vi "Set_Sweep_Frequency.vi"(8 "error in (no error)":errorcluster, 9 "endfreq":dbl, 10 "startfreq":dbl, 11 ".NET Reference in":refnum<k24>) -> (0 "error out":errorcluster, 3 "Reference out":refnum<k24>)   [LabVIEW 2017]
uses:
  D:/test/FULLband-sts/Fullband_Sample/DLL/InstrumentDLL.dll
  DLL/InstrumentDLL.dll
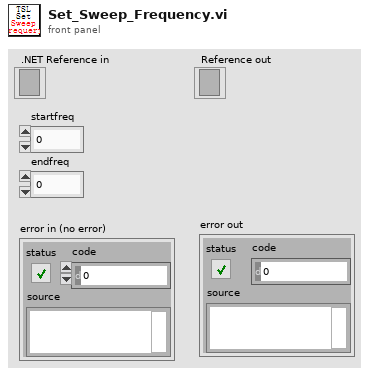
[diagram p1: front panel]
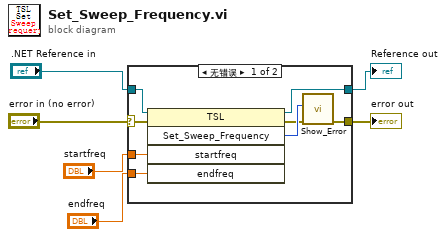
[diagram p0: block diagram]
diagram:
  n1 = case shown="无错误" "error in (no error)" {
    selector: "error in (no error)" -> [w7 w16]
    tunnel: ".NET Reference in" -> [w14 w15]
    tunnel: [w13 w15] -> w5
    tunnel: [w8 w16] -> w4
    tunnel: "startfreq" -> [w12 _]
    tunnel: "endfreq" -> [w11 _]
    frame No Error {
      n2 = invoke on="调用节点" class="TSL" method="Set_Sweep_Frequency"(reference=w14, error in=w7, "startfreq"=w12, "endfreq"=w11) -> (reference out=w13:refnum<k24>, error out=w9:errorcluster, "Set_Sweep_Frequency"=w10:i32)  [unwired: 1 in, 2 out]
      n3 = call "Show_Error.vi"("error in (no error)"=w9, "Error"=w10) -> ("error out"=w8:errorcluster)  [unwired: 9 in]
    }
    frame Error {
    }
  }
  "Reference out" <- w5
  "error out" <- w4
